vi "Process.vi"(8 "error in":errorcluster, 11 "SynchIO.USB4431":refnum<class "SynchIO.PXI-4461.lvclass">) -> (0 "error out":errorcluster, 3 "SynchIO.USB4431 out":refnum<class "SynchIO.PXI-4461.lvclass">)   [LabVIEW 2016, in "SynchIO.PXI-4461.lvclass"]
doc: "---------------------------------------------------------------\nJKI State Machine Objects™\nhttp://jki.net/state-machine-objects/\nCopyright (C) 2005-2015, JKI <info@jki.net>\nALL RIGHTS RESERVEDJKI State Machine Objects (SMO) 1.0.0.5\nJKI - JKI\nCopyright (c) 2016, JKI"
uses:
  SynchIO.PXI-4461.lvclass
  C:/Program Files/National Instruments/LabVIEW 2016/vi.lib/JKI/JKI SMO/SMO/SMO.lvclass
  <vilib>/JKI/JKI SMO/SMO/Typedefs/Parent Call--Enum.ctl
  SynchIO/SynchIO.lvclass
  <vilib>/JKI/JKI SMO/SMO/SMO.lvclass
  <resource>/objmgr/ni.dex.rc
panel:
  in  "Start":bool
  in  "stop":bool
  in  "Tab Control":T1(tab)
  in  "AI Configuration":T2(array[cluster])=[{"AI.Coupling"=enum."DC", "AI.Max"=1.0, "AI.Min"=-1.0, "Input physical channels"="PXI1Slot2/ai0:1"}, {"AI.Coupling"=enum."DC", "AI.Max"=1.0, "AI.Min"=-1.0, "Input physical channels"="PXI1Slot5/ai0:1"}, {"AI.Coupling"=enum."DC", "AI.Max"=1.0, "AI.Min"=-1.0, "Input physical channels"="PXI1Slot6/ai0:1"}]
  in  "AO Configuration":T3(array[cluster])=[{"Output physical channels"="PXI1Slot2/ao0:1", "AO. Max"=1.0, "AO.Min"=-1.0}, {"Output physical channels"="PXI1Slot5/ao0:1", "AO. Max"=1.0, "AO.Min"=-1.0}, {"Output physical channels"="PXI1Slot6/ao0:1", "AO. Max"=1.0, "AO.Min"=-1.0}]
  in  "sampling info":cluster{"Fs":dbl, "#s":dbl}={"Fs"=102388.0, "#s"=7876.0}
  in  "AI Buffer Size (S)":i32=100
  in  "AO":T4={"AO amp (V)"=[1.0, 0.0, 0.0, 0.0, 0.0, 0.0, 0.0, 0.0], "AO DC (V)"=[0.0, 0.0, 0.0, 0.0, 0.0, 0.0, 0.0, 0.0], "AO f (Hz)"=[13.0, 13.0, 13.0, 13.0, 13.0, 13.0, 13.0, 13.0], "AO phi (deg)"=[0.0, 0.0, 0.0, 0.0, 0.0, 0.0, 0.0, 0.0], "function"=[enum."Sine Wave", enum."Sine Wave", enum."Sine Wave", enum."Sine Wave", enum."Sine Wave", enum."Sine Wave", enum."Sine Wave", enum."Sine Wave"]} {"AO DC (V)" format="%#_6p"; "AO amp (V)" format="%#_6p"}
  out "Signals Graph":waveform(dbl)[](graph)=[{"t0"=timestamp(3565974471.4961195 s since 1904-01-01), "dt"=1.0, "Y"=array[6023 elements], "attributes"=variant("NI_ChannelName"=variant(string "Dev2/ai0"), "NI_UnitDescription"=variant(string "Volts"))}, {"t0"=timestamp(3565974471.4961195 s since 1904-01-01), "dt"=1.0, "Y"=array[6023 elements], "attributes"=variant("NI_ChannelName"=variant(string "Dev2/ai1"), "NI_UnitDescription"=variant(string "Volts"))}, {"t0"=timestamp(3565974471.4961195 s since 1904-01-01), "dt"=1.0, "Y"=array[6023 elements], "attributes"=variant("NI_ChannelName"=variant(string "Dev2/ai2"), "NI_UnitDescription"=variant(string "Volts"))}, {"t0"=timestamp(3565974471.4961195 s since 1904-01-01), "dt"=1.0, "Y"=array[6023 elements], "attributes"=variant("NI_ChannelName"=variant(string "Dev2/ai3"), "NI_UnitDescription"=variant(string "Volts"))}, {"t0"=timestamp(3565974471.554943 s since 1904-01-01), "dt"=1.0, "Y"=array[6023 elements], "attributes"=variant("NI_ChannelName"=variant(string "Dev2/ai0"), "NI_UnitDescription"=variant(string "Volts"))}, {"t0"=timestamp(3565974471.554943 s since 1904-01-01), "dt"=1.0, "Y"=array[6023 elements], "attributes"=variant("NI_ChannelName"=variant(string "Dev2/ai1"), "NI_UnitDescription"=variant(string "Volts"))}]
  out "Signals Graph 2":waveform(dbl)[](graph)=[{"t0"=timestamp(3565974471.4961195 s since 1904-01-01), "dt"=1.0, "Y"=array[6023 elements], "attributes"=variant("NI_ChannelName"=variant(string "Dev2/ai0"), "NI_UnitDescription"=variant(string "Volts"))}, {"t0"=timestamp(3565974471.4961195 s since 1904-01-01), "dt"=1.0, "Y"=array[6023 elements], "attributes"=variant("NI_ChannelName"=variant(string "Dev2/ai1"), "NI_UnitDescription"=variant(string "Volts"))}, {"t0"=timestamp(3565974471.4961195 s since 1904-01-01), "dt"=1.0, "Y"=array[6023 elements], "attributes"=variant("NI_ChannelName"=variant(string "Dev2/ai2"), "NI_UnitDescription"=variant(string "Volts"))}, {"t0"=timestamp(3565974471.4961195 s since 1904-01-01), "dt"=1.0, "Y"=array[6023 elements], "attributes"=variant("NI_ChannelName"=variant(string "Dev2/ai3"), "NI_UnitDescription"=variant(string "Volts"))}, {"t0"=timestamp(3565974471.554943 s since 1904-01-01), "dt"=1.0, "Y"=array[6023 elements], "attributes"=variant("NI_ChannelName"=variant(string "Dev2/ai0"), "NI_UnitDescription"=variant(string "Volts"))}, {"t0"=timestamp(3565974471.554943 s since 1904-01-01), "dt"=1.0, "Y"=array[6023 elements], "attributes"=variant("NI_ChannelName"=variant(string "Dev2/ai1"), "NI_UnitDescription"=variant(string "Volts"))}]
  out "Current State":string="Exit"
  out "State History":string
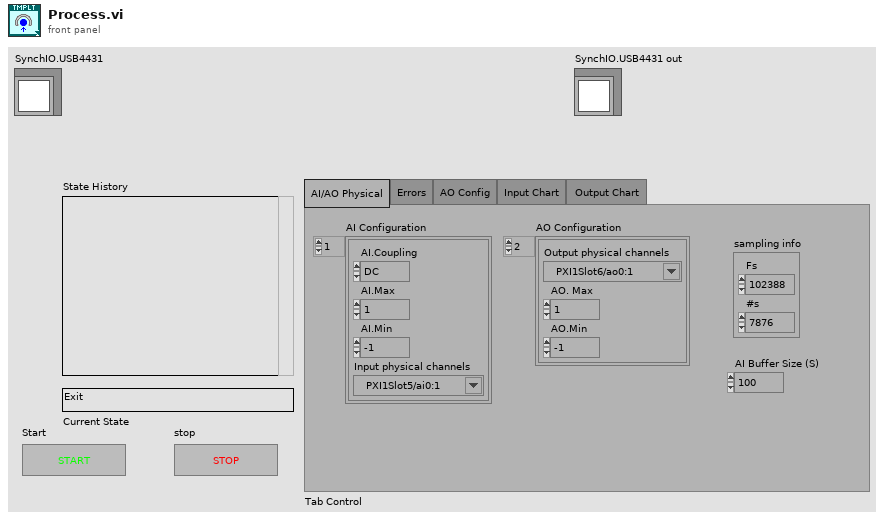
[diagram p1: front panel]
types:
  T1 = enum32{"AI/AO Physical", "Errors", "AO Config", "Input Chart", "Output Chart "}
  T2 = cluster{"AI.Coupling":enum16{"AC", "DC", "GND"}, "AI.Max":dbl, "AI.Min":dbl, "Input physical channels":tag}[]
  T3 = cluster{"Output physical channels":tag, "AO. Max":dbl, "AO.Min":dbl}[]
  T4 = cluster{"AO amp (V)":dbl[], "AO DC (V)":dbl[], "AO f (Hz)":dbl[], "AO phi (deg)":dbl[], "function":enum16{"Sine Wave", "Triangle Wave", "Square Wave", "Sawtooth Wave"}[]}
  T5 = typedef "SMO.lvclass/Parent Call--Enum.ctl" = enum16{"Allows parent to run", "Does not request parent to run"}
  T6 = enum32{"invalid app kind", "Development System", "Run Time System", "Student Edition", "Embedded LabVIEW", "Evaluation", "Custom"}
  T7 = enum32{"Invalid", "Standard", "Closed", "Hidden", "Minimized", "Maximized"}
  T8 = cluster{"Core":cluster{"Current VI Reference":refnum<vi>, "Close Panel on Exit?":bool, "error":errorcluster}, "Self Reference":refnum<class "SynchIO.PXI-4461.lvclass">, "Your string data":string, "AI Buffer Size (S)":i32, "AI Configuration":cluster{"AI.Coupling":enum16{"AC", "DC", "GND"}, "AI.Max":dbl, "AI.Min":dbl, "Input physical channels":tag}[], "AO Configuration":cluster{"Output physical channels":tag, "AO. Max":dbl, "AO.Min":dbl}[], "sampling info":cluster{"Fs":dbl, "#s":dbl}, "AI task":refnum<k21>[], "AO Task":refnum<k21>[], "AI Data":waveform(dbl)[], "AO Data":waveform(dbl)[], "AO":cluster{"AO amp (V)":dbl[], "AO DC (V)":dbl[], "AO f (Hz)":dbl[], "AO phi (deg)":dbl[], "function":enum16{"Sine Wave", "Triangle Wave", "Square Wave", "Sawtooth Wave"}[]}, "Iteration":i32, "writer endpoint":refnum<k21>, "reader endpoint":refnum<k21>, "url":string}
  T9 = cluster{"Current VI Reference":refnum<vi>, "Close Panel on Exit?":bool, "error":errorcluster}
  T10 = typedef "SMO.lvclass/Protected Events.ctl" = cluster{"StopProcesses":refnum<user-event>, "AbortProcesses":refnum<user-event>, "Config Changed":refnum<user-event>, "Dependency":refnum<user-event>}
  T11 = typedef "SynchIO.PXI-4461.lvclass/ProtectedEvents--Cluster.ctl" = cluster{"API_Template":refnum<user-event>}
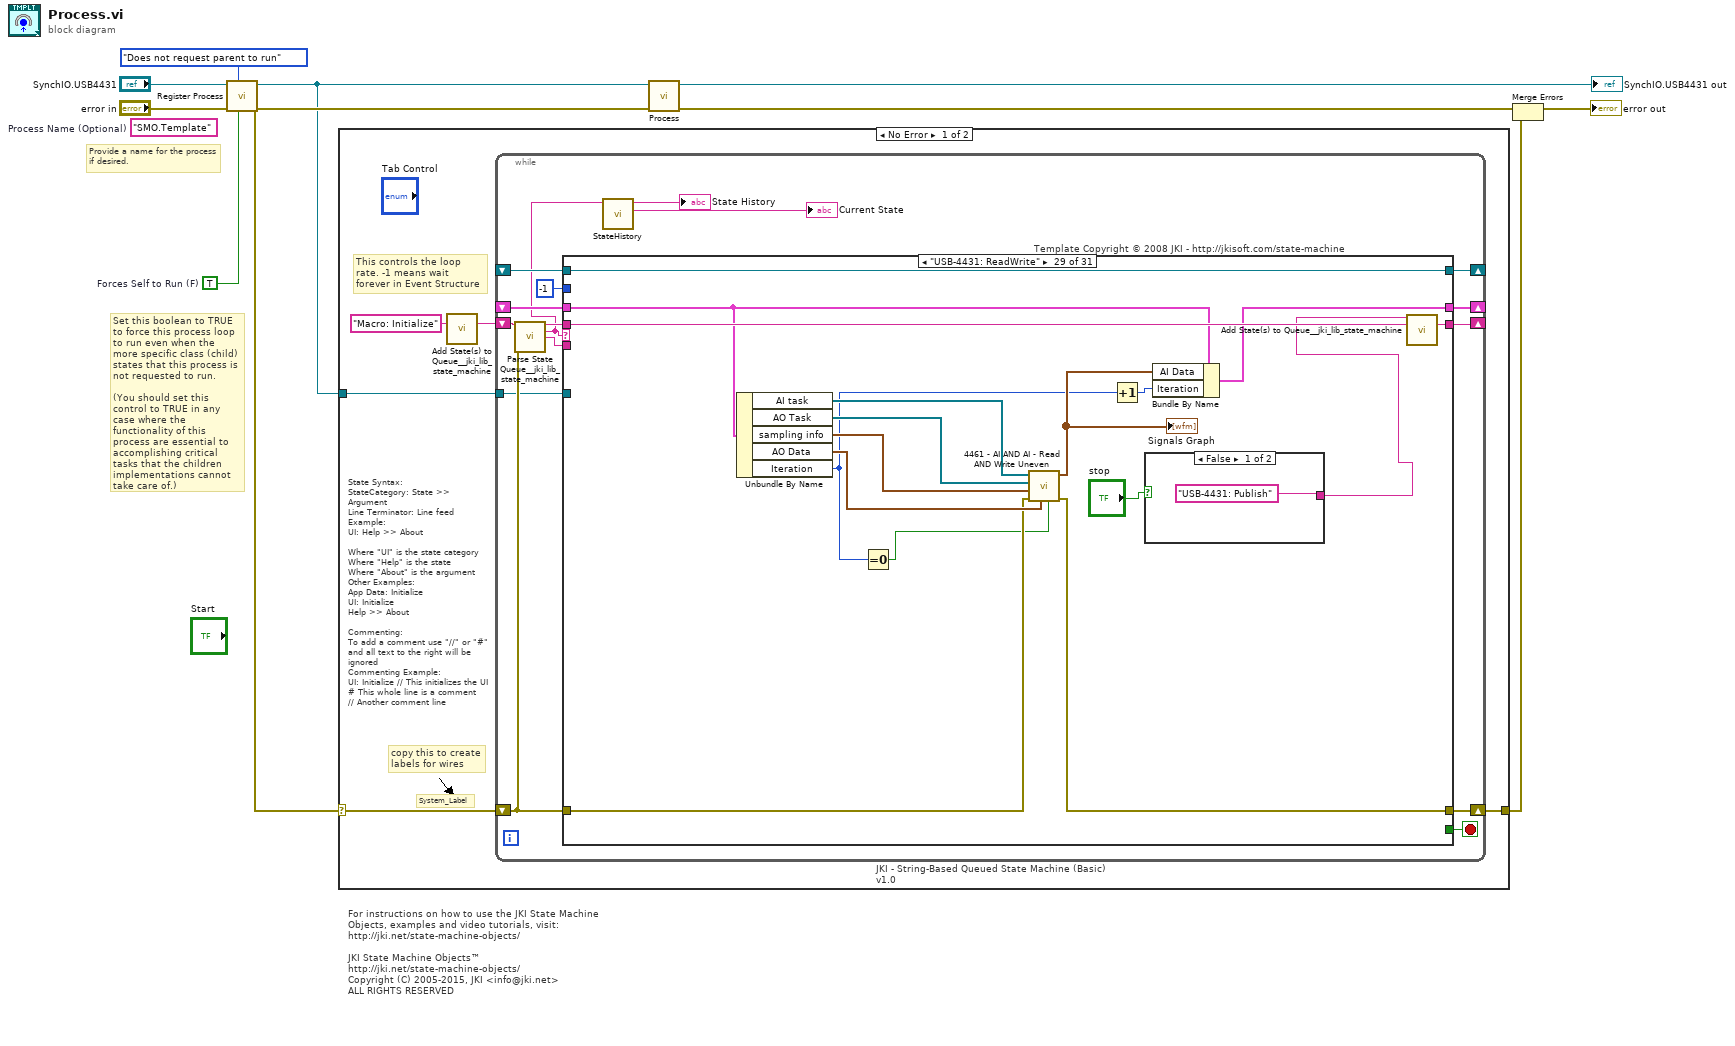
[diagram p0: block diagram]
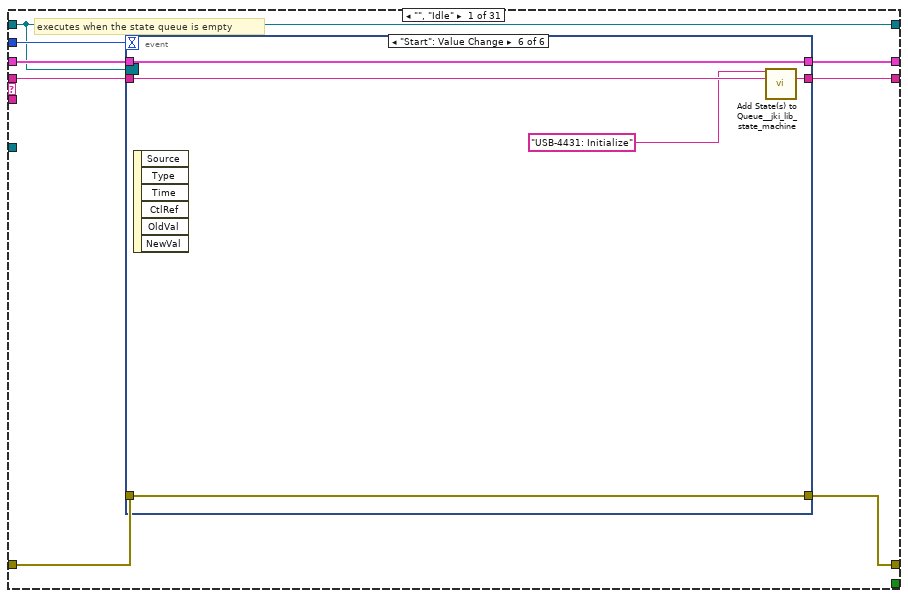
[diagram p2: hidden frame]
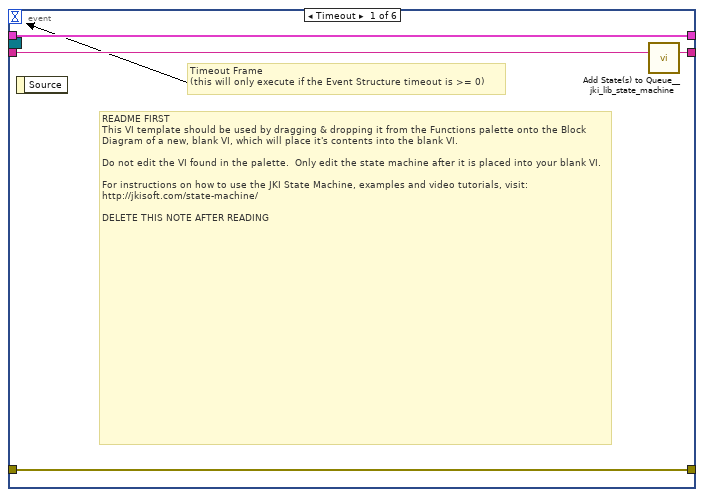
[diagram p3: hidden frame]
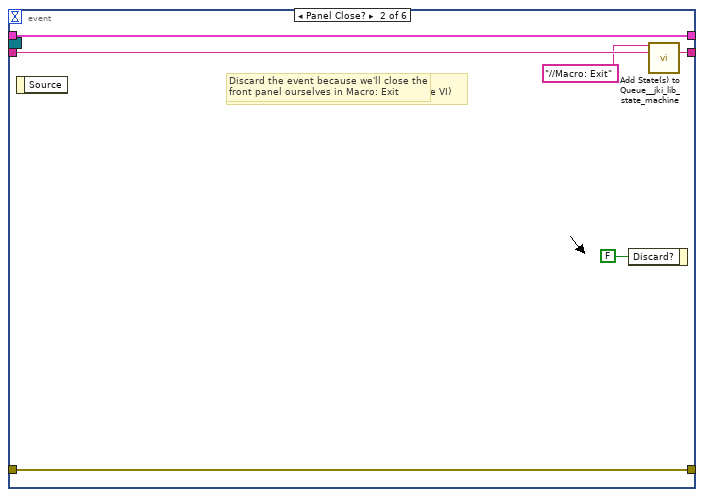
[diagram p4: hidden frame]
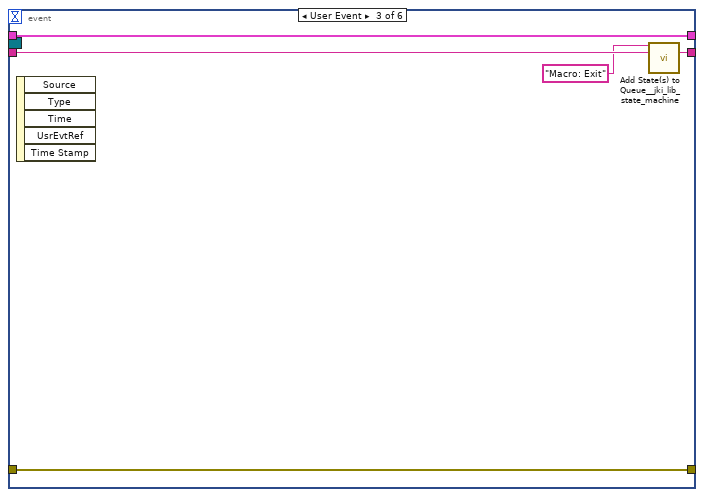
[diagram p5: hidden frame]
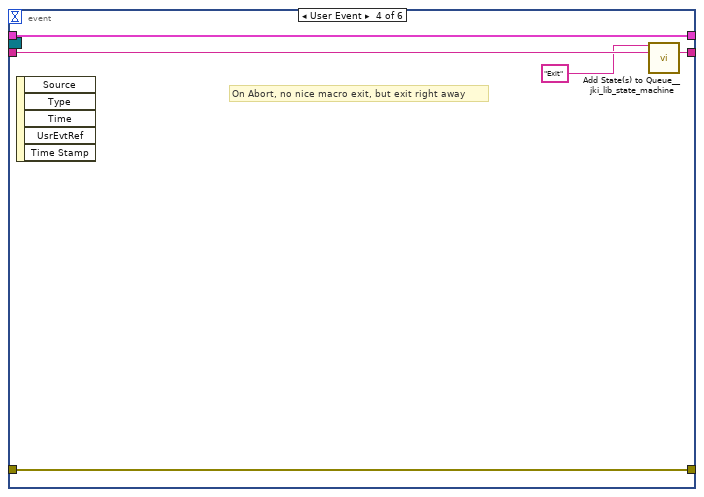
[diagram p6: hidden frame]
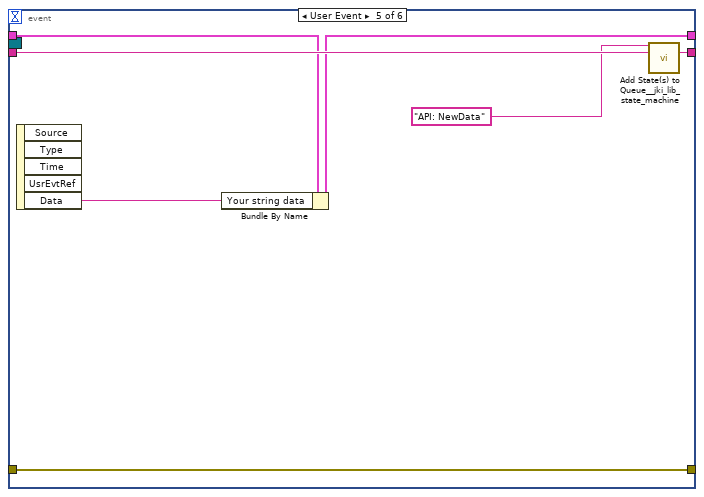
[diagram p7: hidden frame]
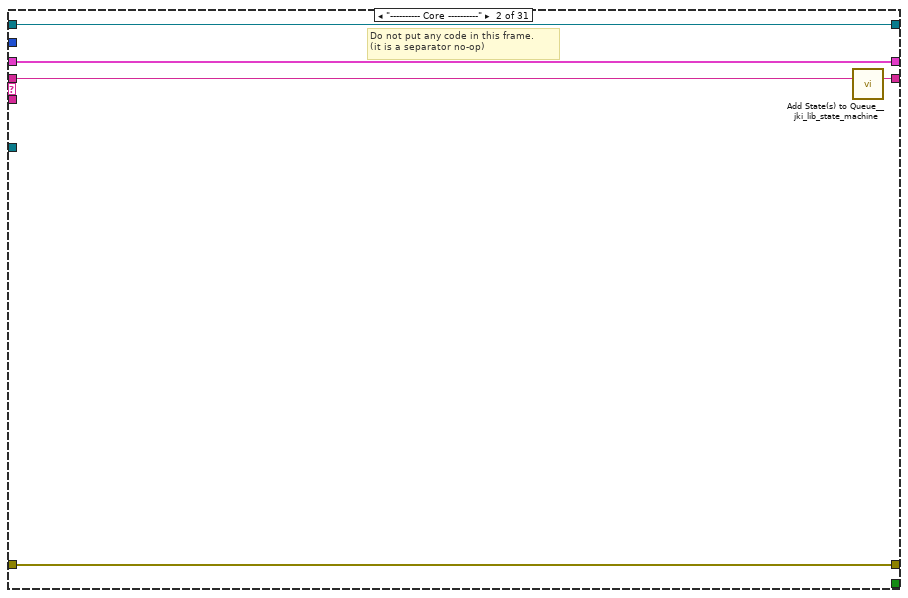
[diagram p8: hidden frame]
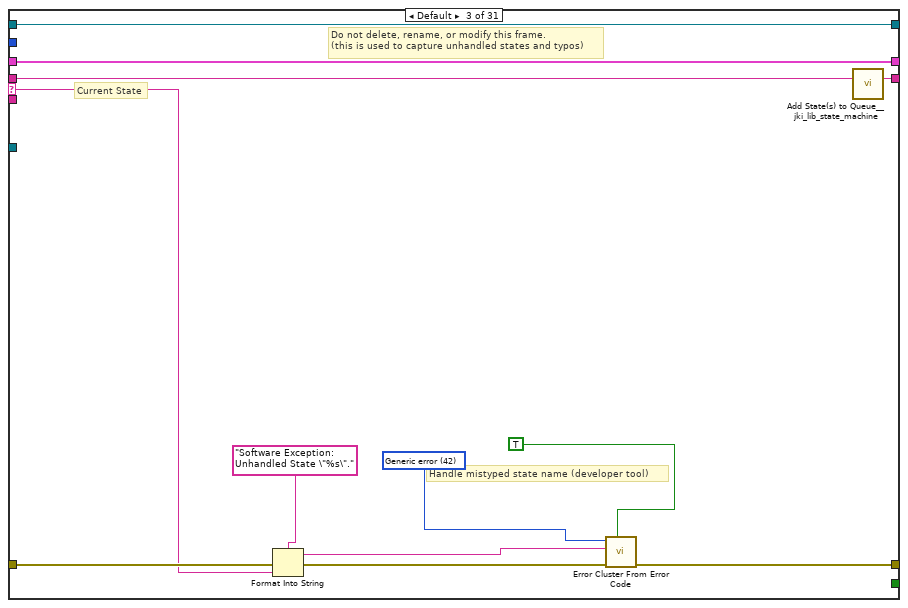
[diagram p9: hidden frame]
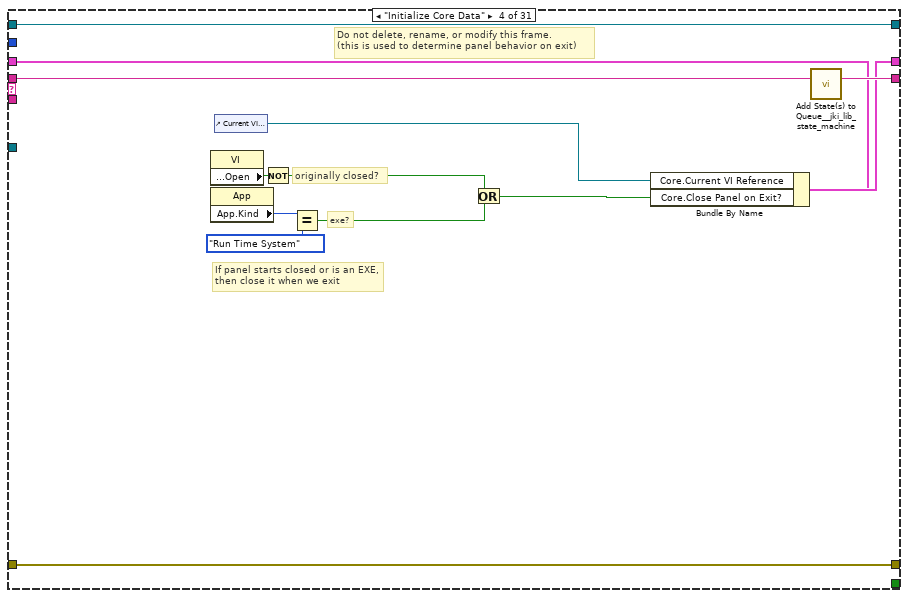
[diagram p10: hidden frame]
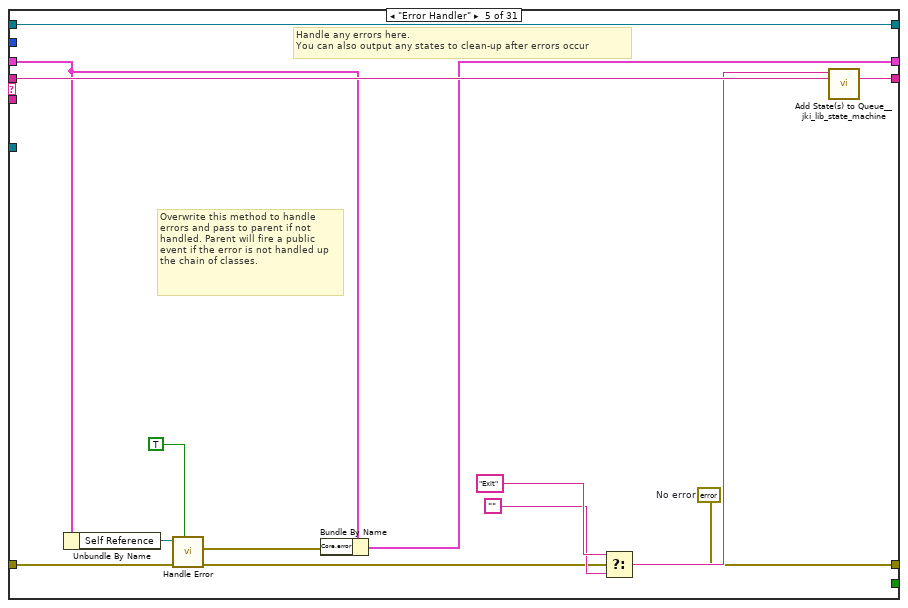
[diagram p11: hidden frame]
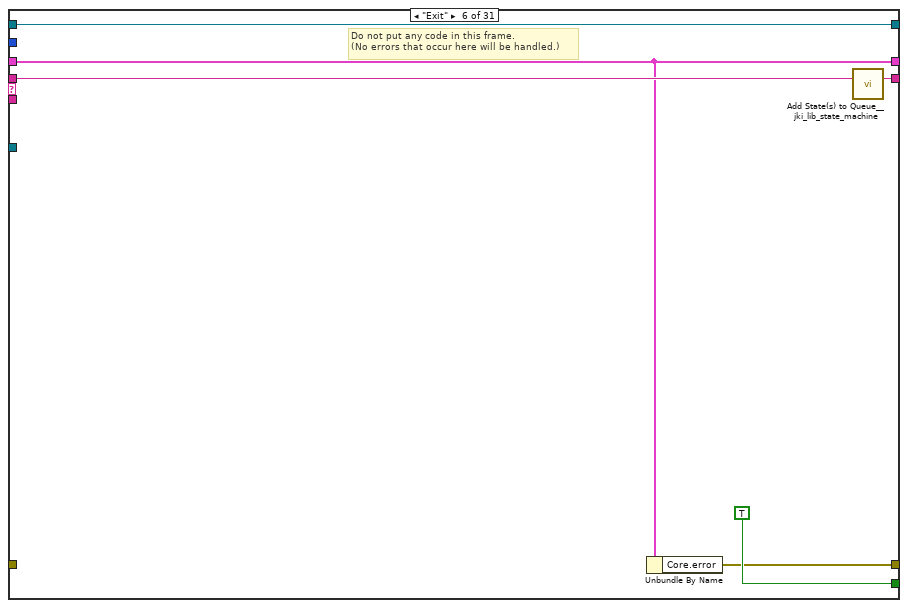
[diagram p12: hidden frame]
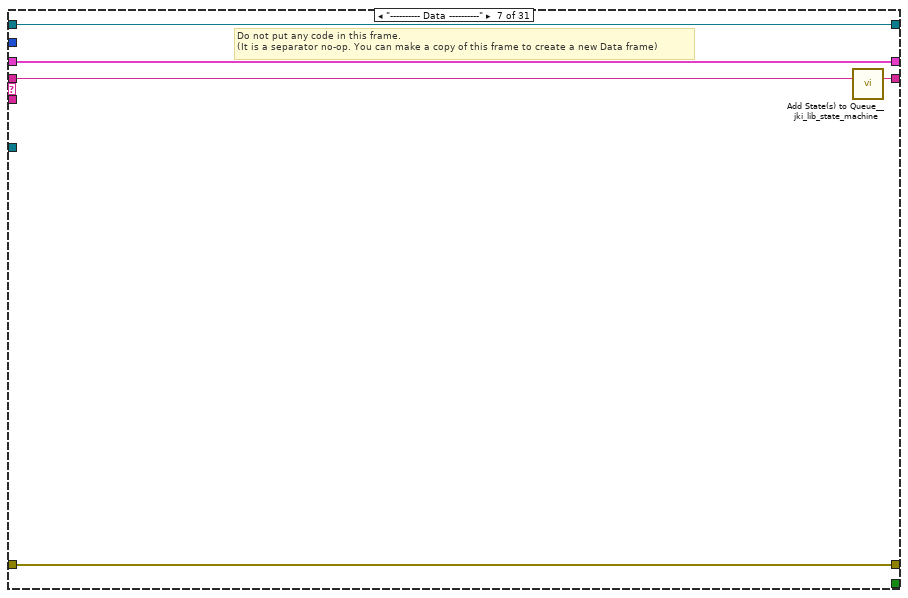
[diagram p13: hidden frame]
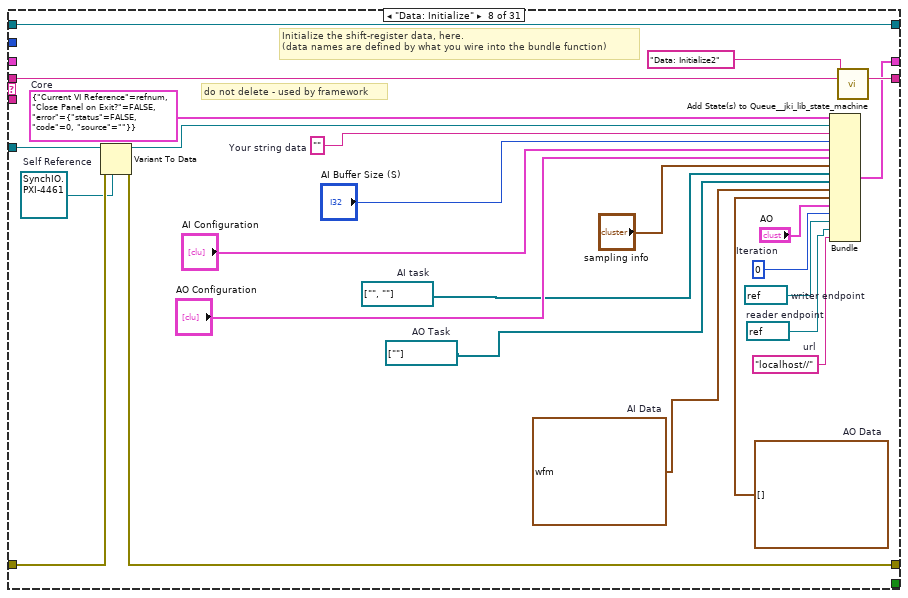
[diagram p14: hidden frame]
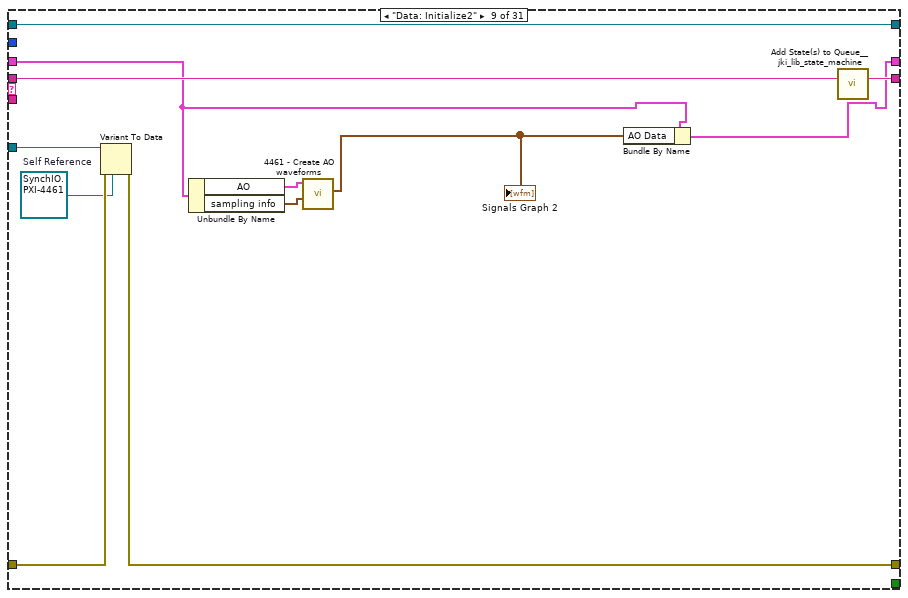
[diagram p15: hidden frame]
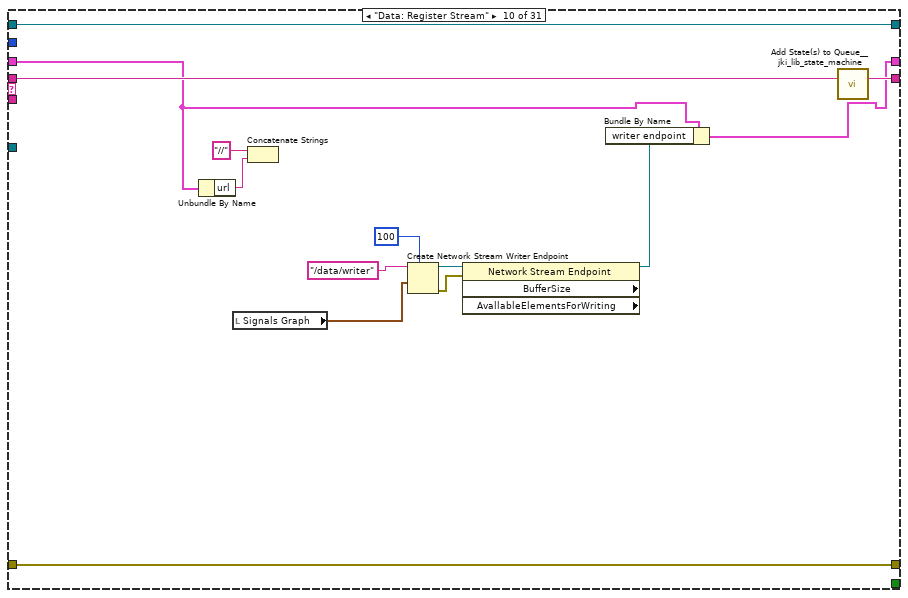
[diagram p16: hidden frame]
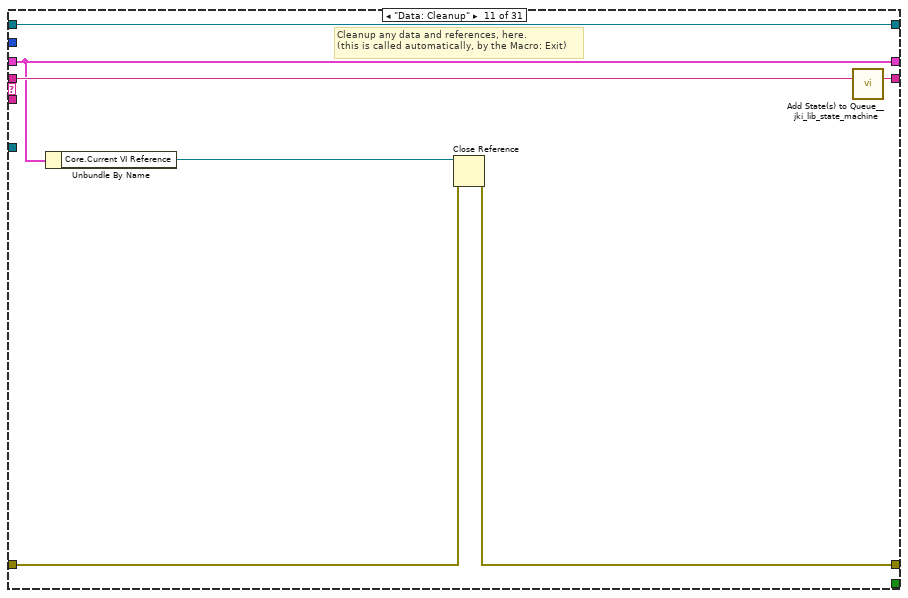
[diagram p17: hidden frame]
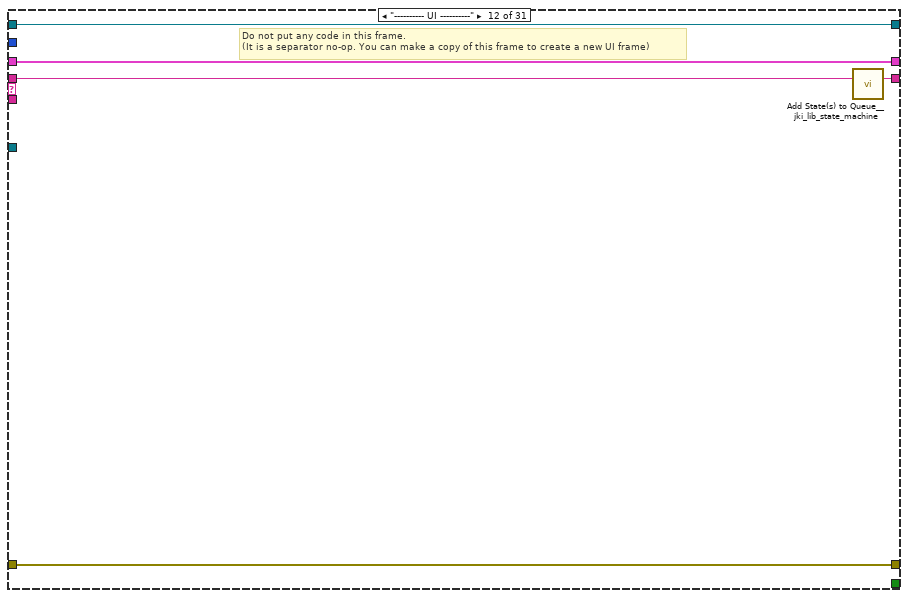
[diagram p18: hidden frame]
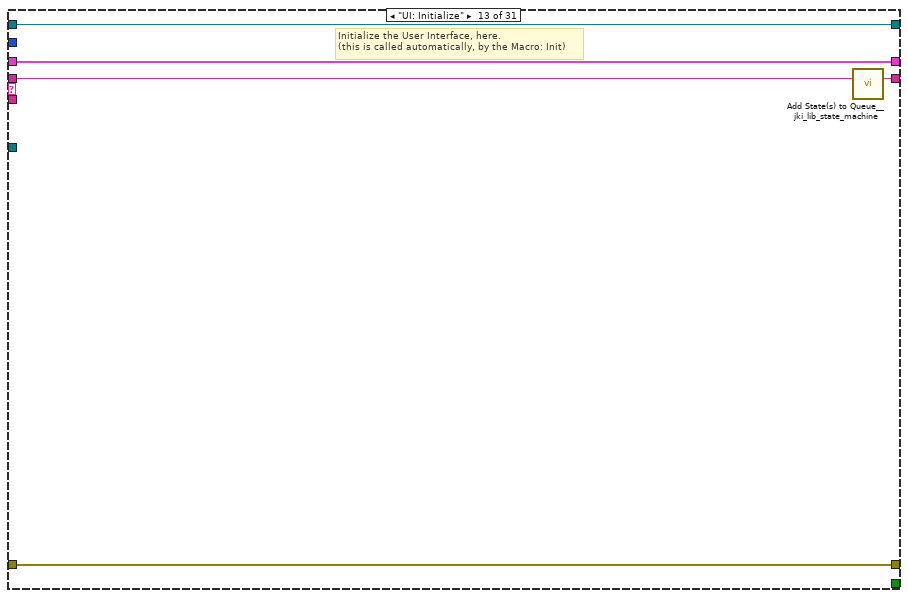
[diagram p19: hidden frame]
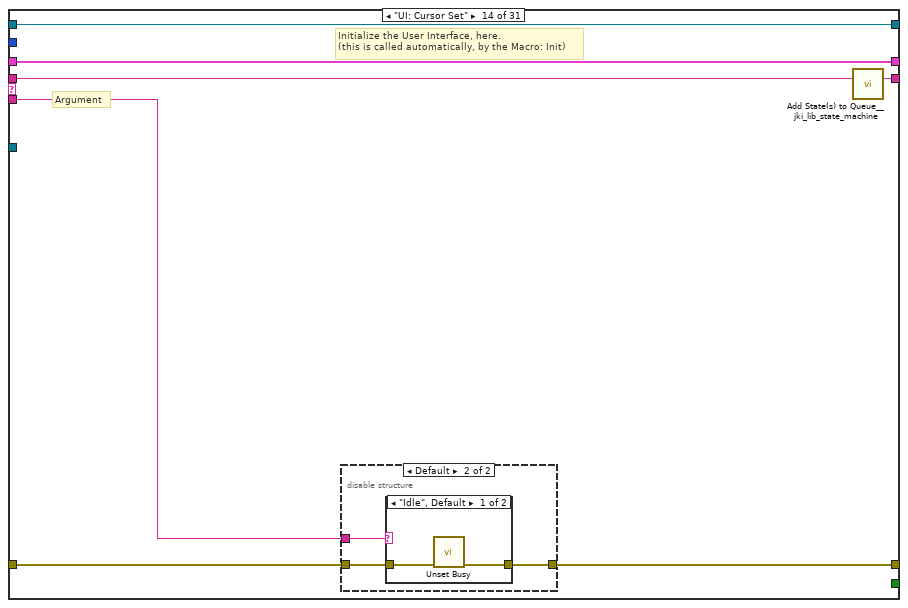
[diagram p20: hidden frame]
diagram:
  w1 = TRUE  # Forces Self to Run (F)
  (unwired) "SMO.Template"  # Process Name (Optional)
  # "Provide a name for the process\nif desired."
  # "Set this boolean to TRUE to force this process loop to run even when the more specific class (child) states that this process is not requested to run.\n\n(You should set this control to TRUE in any case where the functionality of this process are essential to accomplishing critical tasks that the children implementations cannot take care of.)"
  # "For instructions on how to use the JKI State Machine Objects, examples and video tutorials, visit:\nhttp://jki.net/state-machine-objects/\n\nJKI State Machine Objects™\nhttp://jki.net/state-machine-objects/\nCopyright (C) 2005-2015, JKI <info@jki.net>\nALL RIGHTS RESERVED"
  n1 = call <vilib>:"Register Process.vi"("Forces Self to Run (F)"=w1, "Parent Call"=Parent_Call--Enum."Does not request parent to run", "error in (no error)"="error in", "SMO"="SynchIO.USB4431") -> ("error out"=w7:errorcluster, "SMO out"=w6:refnum<class "SynchIO.PXI-4461.lvclass">)  [unwired: 6 in]
  n2 = case shown="No Error" w7 {
    selector: w7 -> [w12 w411]
    tunnel: w6 -> [w13 _]
    tunnel: [w11 w411] -> w3
    frame No Error {
      # "State Syntax:\nStateCategory: State >> Argument\nLine Terminator: Line feed\nExample:\nUI: Help >> About\n\nWhere \"UI\" is the state category\nWhere \"Help\" is the state\nWhere \"About\" is the argument\nOther Examples:\nApp Data: Initialize\nUI: Initialize\nHelp >> About\n\nCommenting:\nTo add a comment use \"//\" or \"#\" and all text to the right will be ignored\nCommenting Example:\nUI: Initialize // This initializes the UI\n# This whole line is a comment\n// Another comment line"
      # "copy this to create labels for wires"
      # "This controls the loop rate. -1 means wait forever in Event Structure"
      # "System_Label"
      n3 = call <vilib>:"Add State(s) to Queue__jki_lib_state_machine.vi"("State(s) in (\"\")"="Macro: Initialize") -> ("States Out"=w15:string)  [unwired: 14 in]
      n4 = while "JKI - String-Based Queued State Machine (Basic) v1.0" {
        shift-right: [w26] -> _
        shift-left: _ -> [w25]
        shift-right: [w29] -> w11
        shift-left: w12 -> [w23]
        shift-right: [w28] -> _
        shift-left: w15 -> [w30]
        tunnel: w13 -> [w22]
        shift-right: [w21] -> _
        shift-left: _ -> [w20]
        stop <- w27 stop-if-true
        # "Template Copyright © 2008 JKI - http://jkisoft.com/state-machine"
        n5 = call <vilib>:"Parse State Queue__jki_lib_state_machine.vi"("State Queue"=w30, "Error In (no error)"=w23) -> ("Remaining States"=w17:string, "Current State"=w16:string, "Arguments"=w31:string)  [unwired: 11 in]
        n6 = case shown="\"USB-4431: ReadWrite\"" w16 {
          selector: w16 -> [_ _ w78 _ _ _ _ _ _ _ _ _ _ _ _ _ _ _ _ _ _ _ _ _ _ _ _ _ _ _ _]
          tunnel: w17 -> [w39 w76 w82 w101 w115 w121 w126 w151 w163 w177 w184 w189 w194 w201 w217 w249 w258 w272 w277 w288 w298 w311 w317 w322 w330 w335 w340 w356 w373 w385 w397]
          tunnel: w31 -> [_ _ _ _ _ _ _ _ _ _ _ _ _ w195 w211 _ _ _ _ _ _ _ _ _ _ _ _ _ _ _ _]
          tunnel: w25 -> [w37 w73 w80 w92 w104 w117 w123 _ w154 w174 w179 w186 w192 w199 w213 w246 w254 w263 w274 w285 w295 w309 w315 w320 w327 w332 w338 w349 w370 w382 w392]
          tunnel: [w36 w74 w84 w98 w106 w116 w124 w146 w160 w167 w180 w187 w191 w196 w214 w247 w256 w270 w275 w279 w296 w299 w313 w318 w324 w331 w336 w345 w365 w379 w394] -> w29
          tunnel: w23 -> [w35 w74 w83 w98 w111 _ w124 w147 w161 w167 w181 w187 w191 w197 w215 w247 w256 w270 w275 w280 w296 w303 w313 w318 w325 w331 w336 w346 w360 w379 w393]
          tunnel: [w38 w75 w81 w100 w114 w120 w125 w150 w162 w176 w183 w188 w193 w200 w216 w248 w257 w271 w276 w287 w297 w310 w316 w321 w329 w334 w339 w355 w372 w384 w396] -> w28
          tunnel: [_ _ _ _ _ TRUE _ _ _ _ _ _ _ _ _ _ _ _ _ _ _ _ _ _ _ _ _ _ _ _ _] -> w27
          tunnel: [w34 w73 w80 w99 w103 w117 w123 w149 w153 w173 w179 w186 w192 w199 w213 w246 w254 w263 w274 w285 w295 w309 w315 w320 w327 w332 w338 w348 w369 w381 w392] -> w26
          tunnel: -1 ("Timeout") -> [w33 _ _ _ _ _ _ _ _ _ _ _ _ _ _ _ _ _ _ _ _ _ _ _ _ _ _ _ _ _ _]
          tunnel: w22 -> [_ _ _ _ _ _ _ w144 w158 _ _ _ _ _ _ _ _ _ _ _ _ _ _ _ _ _ _ _ _ _ _]
          tunnel: [w32 w72 w77 w89 w113 w118 w122 w142 w157 w175 w178 w185 w190 w198 w210 w245 w255 w264 w273 w286 w294 w308 w314 w319 w328 w333 w337 w354 w371 w383 w395] -> w21
          tunnel: w20 -> [w32 w72 w77 w89 w113 w118 w122 w142 w157 w175 w178 w185 w190 w198 w210 w245 w255 w264 w273 w286 w294 _ w314 w319 w328 w333 w337 w354 w371 w383 w395]
          frame "", "Idle" {
            # "executes when the state queue is empty"
            n7 = event shown="[5] \"Start\": Value Change" {
              selector: w32 -> [_ _ _ _ _ _]
              dyn-events: _ -> [_ _ _ _ _ _]
              timeout: w33 -> [_ _ _ _ _ _]
              tunnel: w39 -> [w43 w49 w54 w59 w66 w71]
              tunnel: [w42 w48 w53 w58 w65 w70] -> w38
              tunnel: w37 -> [w40 w46 w51 w56 w63 w67]
              tunnel: [w41 w47 w52 w57 w64 w69] -> w36
              tunnel: w35 -> [w41 w47 w52 w57 w64 w69]
              tunnel: [w40 w46 w51 w56 w62 w67] -> w34
              event Timeout {
                # "README FIRST\nThis VI template should be used by dragging & dropping it from the Functions palette onto the Block Diagram of a new, blank VI, which will place it's contents into the blank VI.\n\nDo not edit the VI found in the palette.  Only edit the state machine after it is placed into your blank VI.\n\nFor instructions on how to use the JKI State Machine, examples and video tutorials, visit:\nhttp://jkisoft.com/state-machine/\n\nDELETE THIS NOTE AFTER READING"
                # "Timeout Frame\n(this will only execute if the Event Structure timeout is >= 0)"
                n8 = event-data() -> ()  [unwired: 1 in, 1 out]
                n9 = call <vilib>:"Add State(s) to Queue__jki_lib_state_machine.vi"("State(s) in (\"\")"=w43) -> ("States Out"=w42:string)  [unwired: 14 in]
              }
              event Panel Close? {
                # "Discard the event because we'll close the front panel ourselves in Macro: Exit"
                # "Close Panel button (pressed) Event\n(this executes Macro: Exit to terminate the VI)"
                n10 = event-data() -> ()  [unwired: 1 in, 1 out]
                n11 = event-data("Discard?"=FALSE) -> ()  [unwired: 1 in, 1 out]
                n12 = call <vilib>:"Add State(s) to Queue__jki_lib_state_machine.vi"("State(s) in Front (\"\")"="//Macro: Exit", "State(s) in (\"\")"=w49) -> ("States Out"=w48:string)  [unwired: 13 in]
              }
              event User Event {
                n13 = event-data() -> ()  [unwired: 1 in, 5 out]
                n14 = call <vilib>:"Add State(s) to Queue__jki_lib_state_machine.vi"("State(s) in Front (\"\")"="Macro: Exit", "State(s) in (\"\")"=w54) -> ("States Out"=w53:string)  [unwired: 13 in]
              }
              event User Event {
                # "On Abort, no nice macro exit, but exit right away"
                n15 = event-data() -> ()  [unwired: 1 in, 5 out]
                n16 = call <vilib>:"Add State(s) to Queue__jki_lib_state_machine.vi"("State(s) in Front (\"\")"="Exit", "State(s) in (\"\")"=w59) -> ("States Out"=w58:string)  [unwired: 13 in]
              }
              event User Event {
                n17 = event-data() -> ("Data"=w60:string)  [unwired: 1 in, 4 out]
                n18 = Bundle By Name(cluster=w63, "Your string data"=w60) -> (w62:T8)
                n19 = call <vilib>:"Add State(s) to Queue__jki_lib_state_machine.vi"("State(s) in Front (\"\")"="API: NewData", "State(s) in (\"\")"=w66) -> ("States Out"=w65:string)  [unwired: 13 in]
              }
              event "Start": Value Change {
                n20 = event-data() -> ()  [unwired: 1 in, 6 out]
                n21 = call <vilib>:"Add State(s) to Queue__jki_lib_state_machine.vi"("State(s) in Front (\"\")"="USB-4431: Initialize", "State(s) in (\"\")"=w71) -> ("States Out"=w70:string)  [unwired: 13 in]
              }
            }
          }
          frame "---------- Core ----------" {
            # "Do not put any code in this frame.\n(it is a separator no-op)"
            n22 = call <vilib>:"Add State(s) to Queue__jki_lib_state_machine.vi"("State(s) in (\"\")"=w76) -> ("States Out"=w75:string)  [unwired: 14 in]
          }
          frame Default {
            w87 = 42 items=["No error", "Argument error", "Memory is full", "Out of zone", "End of file", "File already open", "Generic file I/O error", "File not found", "File permission error", "Disk is full", "Duplicate path", "Too many files open", "System feature not enabled", "Resource file not found", "Cannot add resource", "Resource not found", "Image not found", "Image memory error", "Pen does not exist", "Config type invalid", "Config token not found", "Config parse error", "Config memory error", "Bad external code format", "Bad external code offset", "External code not present", "Null window", "Destroy window error", "Null menu", "Print aborted", "Bad print record", "Print driver error", "Windows error during printing", "Memory error during printing", "Print dialog error", "Generic print error", "Invalid device refnum", "Device not found", "Device parameter error", "Device unit error", "Cannot open device", "Device call aborted", "Generic error", "Cancelled by user", "Object ID too low", "Object ID too high", "Object not in heap", "Unknown heap", "Unknown object (invalid DefProc)", "Unknown object (DefProc not in table)", "Message out of range", "Invalid (null) method", "Unknown message", "Manager call not supported", "Bad address", "Network operation in progress", "Network operation timed out", "Connection is busy", "Network attribute not supported", "Network error", "Address in use", "System out of memory", "Connection aborted", "Connection refused", "Not connected", "Already connected", "Connection closed", "Initialization error (interapplication manager)", "Bad occurrence", "Wait on unbound occurrence handler", "Occurrence queue overflow", "Datalog type conflict", "Unused", "Unrecognized type (interapplication manager)", "Memory corrupt", "Failed to make temporary DLL", "Old CIN version", "Drag socket not found", "Failed to load drop-object", "Failed to register OLE object", "Failed to release OLE object", "Format specifier type mismatch", "Unknown format specifier", "Too few format specifiers", "Too many format specifiers", "Scan failed", "Newer CIN version", "Error converting to variant", "Runtime menu error", "Password tampered", "Variant attribute not found", "Incompatible variant data type", "Event data is not available", "Event Store is not present", "Occurrence is not found", "Event Queue is not created", "Event info is not available", "Refnum passed is NULL", "Error retrieving Class GUID", "Error retrieving CoClass GUID", "Error retrieving TypeLib GUID.", "Bad built application magic bytes.", "Specific driver is different from the specific driver associated with the Logical Name.", "There is no session opened to the class driver.", "Max Error", "MAX - Error with config objects", "MAX - Error loading configuration", "MAX - Group not supported"]
            # "Current State"
            # "Do not delete, rename, or modify this frame.\n(this is used to capture unhandled states and typos)"
            # "Handle mistyped state name (developer tool)"
            n23 = Format Into String(format string="Software Exception: Unhandled State \"%s\"." ("message"), error in=w83, w78) -> (resulting string=w86:string, error out=w85:errorcluster)  [unwired: 1 in]
            n24 = call <vilib>:"Error Cluster From Error Code.vi"("show call chain? (False)"=TRUE, "error in (no error)"=w85, "error message (\"\")"=w86, "error code (0)"=w87) -> ("error out"=w84:errorcluster)  [unwired: 5 in]
            n25 = call <vilib>:"Add State(s) to Queue__jki_lib_state_machine.vi"("State(s) in (\"\")"=w82) -> ("States Out"=w81:string)  [unwired: 14 in]
          }
          frame "Initialize Core Data" {
            # "Do not delete, rename, or modify this frame.\n(this is used to determine panel behavior on exit)"
            # "originally closed?"
            # "exe?"
            # "If panel starts closed or is an EXE, then close it when we exit"
            n26 = property class="VI"() -> ("Front Panel.Open"=w97:bool)  [unwired: 2 in, 2 out]
            n27 = property class="App"() -> ("App.Kind"=w96:T6)  [unwired: 2 in, 2 out]
            n28 = control-ref of="Current VI Reference"() -> (w90:refnum<vi>)
            n29 = Not(x=w97) -> (.not. x?=w94:bool)
            n30 = Equal?(x=w96, y=T6."Run Time System" ("Application:Kind")) -> (x = y?=w93:bool)
            n31 = Or(x=w94, y=w93) -> (x .or. y?=w91:bool)
            n32 = Bundle By Name(cluster=w92, "Core.Current VI Reference"=w90, "Core.Close Panel on Exit?"=w91) -> (w99:T8)
            n33 = call <vilib>:"Add State(s) to Queue__jki_lib_state_machine.vi"("State(s) in (\"\")"=w101) -> ("States Out"=w100:string)  [unwired: 14 in]
          }
          frame "Error Handler" {
            w106 = errorcluster {"status"=FALSE, "code"=0, "source"=""}  # No error
            # "Overwrite this method to handle errors and pass to parent if not handled. Parent will fire a public event if the error is not handled up the chain of classes."
            # "Handle any errors here.\nYou can also output any states to clean-up after errors occur"
            n34 = Unbundle By Name(w104) -> ("Self Reference"=w112:refnum<class "SynchIO.PXI-4461.lvclass">)
            n35 = call-dynamic "Handle Error.vi"("Stop on Unhandled Error (T)"=TRUE, "error in"=w111, "SMO"=w112) -> ("handling error"=w107:errorcluster, "Unhandled error"=w105:errorcluster)  [unwired: 6 in, 1 out]
            n36 = Bundle By Name(cluster=w104, "Core.error"=w105) -> (w103:T8)
            n37 = Select(t="Exit", s=w107, f="") -> (s? t:f=w108:string)
            n38 = call <vilib>:"Add State(s) to Queue__jki_lib_state_machine.vi"("State(s) in Front (\"\")"=w108, "State(s) in (\"\")"=w115) -> ("States Out"=w114:string)  [unwired: 13 in]
          }
          frame "Exit" {
            # "Do not put any code in this frame.\n(No errors that occur here will be handled.)"
            n39 = Unbundle By Name(w117) -> ("Core.error"=w116:errorcluster)
            n40 = call <vilib>:"Add State(s) to Queue__jki_lib_state_machine.vi"("State(s) in (\"\")"=w121) -> ("States Out"=w120:string)  [unwired: 14 in]
          }
          frame "---------- Data ----------" {
            # "Do not put any code in this frame.\n(It is a separator no-op. You can make a copy of this frame to create a new Data frame)"
            n41 = call <vilib>:"Add State(s) to Queue__jki_lib_state_machine.vi"("State(s) in (\"\")"=w126) -> ("States Out"=w125:string)  [unwired: 14 in]
          }
          frame "Data: Initialize" {
            w127 = "localhost//"  # url
            w128 = refnum<k21> refnum  # reader endpoint
            w129 = waveform(dbl)[] [{"t0"=timestamp(3565974471.4961195 s since 1904-01-01), "dt"=1.0, "Y"=array[6023 elements], "attributes"=variant("NI_ChannelName"=variant(string "Dev2/ai0"), "NI_UnitDescription"=variant(string "Volts"))}, {"t0"=timestamp(3565974471.4961195 s since 1904-01-01), "dt"=1.0, "Y"=array[6023 elements], "attributes"=variant("NI_ChannelName"=variant(string "Dev2/ai1"), "NI_UnitDescription"=variant(string "Volts"))}, {"t0"=timestamp(3565974471.4961195 s since 1904-01-01), "dt"=1.0, "Y"=array[6023 elements], "attributes"=variant("NI_ChannelName"=variant(string "Dev2/ai2"), "NI_UnitDescription"=variant(string "Volts"))}, {"t0"=timestamp(3565974471.4961195 s since 1904-01-01), "dt"=1.0, "Y"=array[6023 elements], "attributes"=variant("NI_ChannelName"=variant(string "Dev2/ai3"), "NI_UnitDescription"=variant(string "Volts"))}, {"t0"=timestamp(3565974471.554943 s since 1904-01-01), "dt"=1.0, "Y"=array[6023 elements], "attributes"=variant("NI_ChannelName"=variant(string "Dev2/ai0"), "NI_UnitDescription"=variant(string "Volts"))}, {"t0"=timestamp(3565974471.554943 s since 1904-01-01), "dt"=1.0, "Y"=array[6023 elements], "attributes"=variant("NI_ChannelName"=variant(string "Dev2/ai1"), "NI_UnitDescription"=variant(string "Volts"))}]  # AI Data
            w130 = refnum<k21> refnum  # writer endpoint
            w131 = 0  # Iteration
            w133 = waveform(dbl)[] []  # AO Data
            w134 = refnum<k21>[] [""]  # AO Task
            w135 = refnum<k21>[] ["", ""]  # AI task
            w141 = T9 {"Current VI Reference"=refnum, "Close Panel on Exit?"=FALSE, "error"={"status"=FALSE, "code"=0, "source"=""}}  # Core
            w145 = refnum<class "SynchIO.PXI-4461.lvclass"> refnum  # Self Reference
            w148 = ""  # Your string data
            # "do not delete - used by framework"
            # "Initialize the shift-register data, here.\n(data names are defined by what you wire into the bundle function)"
            n42 = Variant To Data(error in=w147, type=w145, Variant=w144) -> (data=w143:refnum<class "SynchIO.PXI-4461.lvclass">, error out=w146:errorcluster)
            n43 = Bundle("Core"=w141, "Self Reference"=w143, "Your string data"=w148, "AI Buffer Size (S)"="AI Buffer Size (S)", "AI Configuration"="AI Configuration", "AO Configuration"="AO Configuration", "sampling info"="sampling info", "AI task"=w135, "AO Task"=w134, "AI Data"=w129, "AO Data"=w133, "AO"="AO", "Iteration"=w131, "writer endpoint"=w130, "reader endpoint"=w128, "url"=w127) -> (w149:T8)  [unwired: 1 in]
            n44 = call <vilib>:"Add State(s) to Queue__jki_lib_state_machine.vi"("State(s) in Front (\"\")"="Data: Initialize2" ("State(s) in Front (\"\")"), "State(s) in (\"\")"=w151) -> ("States Out"=w150:string)  [unwired: 13 in]
          }
          frame "Data: Initialize2" {
            w159 = refnum<class "SynchIO.PXI-4461.lvclass"> refnum  # Self Reference
            n45 = Variant To Data(error in=w161, type=w159, Variant=w158) -> (error out=w160:errorcluster)  [unwired: 1 out]
            n46 = Unbundle By Name(w154) -> ("AO"=w155:T4, "sampling info"=w156:cluster{"Fs":dbl, "#s":dbl})
            n47 = call "4461 - Create AO waveforms.vi"("sampling info"=w156, "AO"=w155) -> ("AO Array"=w152:waveform(dbl)[])  [unwired: 6 in, 3 out]
            "Signals Graph 2" <- w152
            n48 = Bundle By Name(cluster=w154, "AO Data"=w152) -> (w153:T8)
            n49 = call <vilib>:"Add State(s) to Queue__jki_lib_state_machine.vi"("State(s) in (\"\")"=w163) -> ("States Out"=w162:string)  [unwired: 14 in]
          }
          frame "Data: Register Stream" {
            n50 = Unbundle By Name(w174) -> ("url"=w164:string)
            n51 = local read "Signals Graph"() -> (w166:waveform(dbl)[])
            n52 = Concatenate Strings("//" ("reader url"), w164) -> ()  [unwired: 1 out]
            n53 = Create Network Stream Writer Endpoint(7:100 ("writer buffer size"), 9:w166, 11:"/data/writer" ("reader url")) -> (0:w170:errorcluster, 3:w171:refnum<k21>)  [unwired: 4 in]
            n54 = property class="Network Stream Endpoint" props=["BufferSize", "AvallableElementsForWriting"](reference=w171, error in=w170) -> (reference out=w168:refnum<k21>)  [unwired: 3 out]
            n55 = Bundle By Name(cluster=w174, "writer endpoint"=w168) -> (w173:T8)
            n56 = call <vilib>:"Add State(s) to Queue__jki_lib_state_machine.vi"("State(s) in (\"\")"=w177) -> ("States Out"=w176:string)  [unwired: 14 in]
          }
          frame "Data: Cleanup" {
            # "Cleanup any data and references, here.\n(this is called automatically, by the Macro: Exit)"
            n57 = Unbundle By Name(w179) -> ("Core.Current VI Reference"=w182:refnum<vi>)
            n58 = Close Reference(reference=w182, error in (no error)=w181) -> (error out=w180:errorcluster)
            n59 = call <vilib>:"Add State(s) to Queue__jki_lib_state_machine.vi"("State(s) in (\"\")"=w184) -> ("States Out"=w183:string)  [unwired: 14 in]
          }
          frame "---------- UI ----------" {
            # "Do not put any code in this frame.\n(It is a separator no-op. You can make a copy of this frame to create a new UI frame)"
            n60 = call <vilib>:"Add State(s) to Queue__jki_lib_state_machine.vi"("State(s) in (\"\")"=w189) -> ("States Out"=w188:string)  [unwired: 14 in]
          }
          frame "UI: Initialize" {
            # "Initialize the User Interface, here.\n(this is called automatically, by the Macro: Init)"
            n61 = call <vilib>:"Add State(s) to Queue__jki_lib_state_machine.vi"("State(s) in (\"\")"=w194) -> ("States Out"=w193:string)  [unwired: 14 in]
          }
          frame "UI: Cursor Set" {
            # "Argument"
            # "Initialize the User Interface, here.\n(this is called automatically, by the Macro: Init)"
            n62 = disable-structure shown="Default" {
              disable-tunnel: w197 -> [w202 w205]
              disable-tunnel: [w202 w204] -> w196
              disable-tunnel: w195 -> [_ w203]
              frame condition #0 {
              }
              frame condition #1 (active) {
                n63 = case shown="\"Idle\", Default" w203 {
                  tunnel: w205 -> [w207 w209]
                  tunnel: [w206 w208] -> w204
                  frame "Idle", Default {
                    n64 = call <vilib>:"Unset Busy.vi"("error in (no error)"=w207) -> ("error out"=w206:errorcluster)  [unwired: 10 in]
                  }
                  frame "Busy" {
                    n65 = call <vilib>:"Set Busy.vi"("error in (no error)"=w209) -> ("error out"=w208:errorcluster)  [unwired: 9 in, 1 out]
                  }
                }
              }
            }
            n66 = call <vilib>:"Add State(s) to Queue__jki_lib_state_machine.vi"("State(s) in (\"\")"=w201) -> ("States Out"=w200:string)  [unwired: 14 in]
          }
          frame "UI: Front Panel State" {
            # "Argument"
            # "Set Front Panel Open or Closed\n(Usage: \"UI: Front Panel State >> Open|Close\")"
            n67 = Unbundle By Name(w213) -> ("Core.Current VI Reference"=w212:refnum<vi>)
            n68 = disable-structure shown="Default" {
              disable-tunnel: w215 -> [w221 w244]
              disable-tunnel: [w220 w244] -> w214
              disable-tunnel: w212 -> [w219 _]
              disable-tunnel: w211 -> [w218 _]
              frame condition #0 (active) {
                n69 = case shown="\"Open\", Default" w218 {
                  tunnel: w221 -> [w225 w238]
                  tunnel: [w227 w239] -> w220
                  tunnel: w219 -> [w226 w236]
                  frame "Open", Default {
                    n70 = property class="VI"(reference=w226, error in=w225) -> (reference out=w223:refnum<vi>, error out=w224:errorcluster, "FP.State"=w222:T7)
                    n71 = case shown="\"Closed\"" w222 {
                      tunnel: [w230 w233] -> w227
                      tunnel: w224 -> [w229 w233]
                      tunnel: w223 -> [w228 _]
                      frame "Closed" {
                        n72 = invoke class="VI" method="FP.Open"(reference=w228, error in=w229, "Activate"=TRUE, "State"=T7."Standard") -> (error out=w230:errorcluster)  [unwired: 1 in, 4 out]
                      }
                      frame Default {
                      }
                    }
                  }
                  frame "Close" {
                    n73 = property class="VI"(reference=w236, error in=w238) -> (reference out=w235:refnum<vi>, error out=w237:errorcluster, "FP.State"=w234:T7)
                    n74 = case shown="Default" w234 {
                      tunnel: [w240 w243] -> w239
                      tunnel: w237 -> [w240 w242]
                      tunnel: w235 -> [_ w241]
                      frame "Invalid", "Closed" {
                      }
                      frame Default {
                        n75 = invoke class="VI" method="FP.Close"(reference=w241, error in=w242) -> (error out=w243:errorcluster)  [unwired: 1 in, 2 out]
                      }
                    }
                  }
                }
              }
              frame condition #1 {
              }
            }
            n76 = call <vilib>:"Add State(s) to Queue__jki_lib_state_machine.vi"("State(s) in (\"\")"=w217) -> ("States Out"=w216:string)  [unwired: 14 in]
          }
          frame "---------- Macro ----------" {
            # "Do not put any code in this frame.\n(It is a separator no-op. You can make a copy of this frame to create a new Macro frame)"
            n77 = call <vilib>:"Add State(s) to Queue__jki_lib_state_machine.vi"("State(s) in (\"\")"=w249) -> ("States Out"=w248:string)  [unwired: 14 in]
          }
          frame "Macro: Initialize" {
            # "Initialization Macro\n(This is called once, when the VI starts)"
            n78 = call <vilib>:"Add State(s) to Queue__jki_lib_state_machine.vi"("State(s) in Front (\"\")"="Data: Initialize\nInitialize Core Data\nEvents: Register", "State(s) in (\"\")"="Process: Sync", "State(s) at Back (\"\")"="UI: Initialize\nUI: Front Panel State >> Open\nData: Register Stream") -> ("States Out"=w251:string)  [unwired: 12 in]
            n79 = call <vilib>:"Add State(s) to Queue__jki_lib_state_machine.vi"("State(s) in Front (\"\")"=w251, "State(s) in (\"\")"=w258) -> ("States Out"=w257:string)  [unwired: 13 in]
          }
          frame "Macro: Exit" {
            # "Exit Macro\n(This is called once, when the VI exits)"
            n80 = Unbundle By Name(w263) -> ("Core.Close Panel on Exit?"=w269:bool)
            n81 = Select(t="//UI: Front Panel State >> Close", s=w269, f="") -> (s? t:f=w266:string)
            n82 = call <vilib>:"Add State(s) to Queue__jki_lib_state_machine.vi"("State(s) in Front (\"\")"="USB4431: Shutdown\nData: Cleanup\nEvents: Unregister", "State(s) in (\"\")"="Process: Sync", "State(s) at Back (\"\")"="Exit") -> ("States Out"=w260:string)  [unwired: 12 in]
            n83 = call <vilib>:"Add State(s) to Queue__jki_lib_state_machine.vi"("State(s) in (\"\")"=w266, "State(s) at Back (\"\")"=w260) -> ("States Out"=w265:string)  [unwired: 13 in]
            n84 = call <vilib>:"Add State(s) to Queue__jki_lib_state_machine.vi"("State(s) in Front (\"\")"=w265, "State(s) in (\"\")"=w272) -> ("States Out"=w271:string)  [unwired: 13 in]
          }
          frame "---------- Process ----------" {
            # "Template Separator\n(You can make a copy of, or modify, this frame)"
            n85 = call <vilib>:"Add State(s) to Queue__jki_lib_state_machine.vi"("State(s) in (\"\")"=w277) -> ("States Out"=w276:string)  [unwired: 14 in]
          }
          frame "Process: Sync" {
            n86 = Unbundle By Name(w285) -> ("Self Reference"=w281:refnum<class "SynchIO.PXI-4461.lvclass">)
            n87 = disable-structure shown="Enabled" {
              disable-tunnel: [w292 FALSE ("Don't run?")] -> w284
              disable-tunnel: w281 -> [w291 _]
              disable-tunnel: w280 -> [w290 _]
              disable-tunnel: [w289 _] -> w279
              frame Enabled {
                n88 = call <vilib>:"WaitOnProcessSync.vi"("error in (no error)"=w290, "SMO"=w291) -> ("error out"=w289:errorcluster, "Don't run?"=w292:bool)  [unwired: 7 in, 1 out]
              }
              frame Disabled {
              }
            }
            n89 = Select(t="Data: Cleanup\nEvents: Unregister\nExit", s=w284, f="") -> (s? t:f=w278:string)
            n90 = call <vilib>:"Add State(s) to Queue__jki_lib_state_machine.vi"("State(s) in Front (\"\")"=w278, "State(s) in (\"\")"=w288) -> ("States Out"=w287:string)  [unwired: 13 in]
          }
          frame "---------- Events ----------" {
            # "Template Separator\n(You can make a copy of, or modify, this frame)"
            n91 = call <vilib>:"Add State(s) to Queue__jki_lib_state_machine.vi"("State(s) in (\"\")"=w298) -> ("States Out"=w297:string)  [unwired: 14 in]
          }
          frame "Events: Register" {
            # "Expand to add\nmore events"
            # "Self Events (API Calls)"
            # "Base Class Protected Events"
            n92 = Unbundle By Name(w309) -> ("Self Reference"=w304:refnum<class "SynchIO.PXI-4461.lvclass">)
            n93 = call <vilib>:"GetProtectedEvents.vi"("SMO"=w304) -> ("error out"=w300:errorcluster, "SMO Protected Events"=w307:T10, "SMO out"=w306:refnum<class "SynchIO.PXI-4461.lvclass">)  [unwired: 8 in]
            n94 = call "SynchIO.USB4431.GetProtectedEvents.vi"("SynchIO.USB4431"=w306) -> ("error out"=w301:errorcluster, "Protected Events"=w305:T11)  [unwired: 8 in, 1 out]
            n95 = register-events(w307, w305) -> (reference out=w308:refnum<event-registration>, error out=w302:errorcluster)  [unwired: 2 in]
            n96 = Merge Errors(w303, w302, w301, w300) -> (w299:errorcluster)
            n97 = call <vilib>:"Add State(s) to Queue__jki_lib_state_machine.vi"("State(s) in (\"\")"=w311) -> ("States Out"=w310:string)  [unwired: 14 in]
          }
          frame "Events: Unregister" {
            n98 = Unregister For Events(event registration refnum=w314, error in=w313) -> (error out=w312:errorcluster)
            n99 = call <vilib>:"Clear Errors.vi"("error in (no error)"=w312) -> ()  [unwired: 5 in, 2 out]
            n100 = call <vilib>:"Add State(s) to Queue__jki_lib_state_machine.vi"("State(s) in (\"\")"=w317) -> ("States Out"=w316:string)  [unwired: 14 in]
          }
          frame "---------- API ----------" {
            n101 = call <vilib>:"Add State(s) to Queue__jki_lib_state_machine.vi"("State(s) in (\"\")"=w322) -> ("States Out"=w321:string)  [unwired: 14 in]
          }
          frame "API: NewData" {
            n102 = Unbundle By Name(w327) -> ("Self Reference"=w326:refnum<class "SynchIO.PXI-4461.lvclass">, "Your string data"=w323:string)
            n103 = call "SynchIO.USB4431.SetData.vi"("error in (no error)"=w325, "Data In"=w323, "SynchIO.USB4431"=w326) -> ("error out"=w324:errorcluster)  [unwired: 7 in, 1 out]
            n104 = call <vilib>:"Add State(s) to Queue__jki_lib_state_machine.vi"("State(s) in (\"\")"=w330, "State(s) at Back (\"\")"=w323) -> ("States Out"=w329:string)  [unwired: 13 in]
          }
          frame "API: Initialize" {
            n105 = call <vilib>:"Add State(s) to Queue__jki_lib_state_machine.vi"("State(s) in (\"\")"=w335) -> ("States Out"=w334:string)  [unwired: 14 in]
          }
          frame "----------USB-4431---------- " {
            n106 = call <vilib>:"Add State(s) to Queue__jki_lib_state_machine.vi"("State(s) in (\"\")"=w340) -> ("States Out"=w339:string)  [unwired: 14 in]
          }
          frame "USB-4431: Initialize" {
            w342 = 10123 items=["Finite Samples"=10178, "Continuous Samples"=10123] ("sample mode")
            n107 = Unbundle By Name(w349) -> ("AI Buffer Size (S)"=w341:i32, "AI Configuration"=w353:T2, "AO Configuration"=w352:T3, "AO"=w351:T4, "sampling info"=w350:cluster{"Fs":dbl, "#s":dbl})
            n108 = call "4461 - Create IO Channels Parallel Uneven.vi"("sample mode"=w342, "error in"=w346, "AI Buffer Size (S)"=w341, "sampling info"=w350, "AO"=w351, "AO Configuration"=w352, "AI Configuration"=w353) -> ("AO Task"=w343:refnum<k21>[], "AI task"=w344:refnum<k21>[], "error out"=w345:errorcluster)  [unwired: 1 in, 1 out]
            n109 = Bundle By Name(cluster=w349, "AI task"=w344, "AO Task"=w343) -> (w348:T8)
            n110 = call <vilib>:"Add State(s) to Queue__jki_lib_state_machine.vi"("State(s) in Front (\"\")"="USB-4431: ReadWrite" ("message"), "State(s) in (\"\")"=w356) -> ("States Out"=w355:string)  [unwired: 13 in]
          }
          frame "USB-4431: ReadWrite" {
            n111 = Unbundle By Name(w370) -> ("AI task"=w363:refnum<k21>[], "AO Task"=w364:refnum<k21>[], "sampling info"=w368:cluster{"Fs":dbl, "#s":dbl}, "AO Data"=w362:waveform(dbl)[], "Iteration"=w357:i32)
            n112 = Equal To 0?(x=w357) -> (x = 0?=w359:bool)
            n113 = call "4461 - AI AND AI - Read AND Write Uneven.vi"("Reset"=w359, "AO Array"=w362, "error in (no error)"=w360, "sampling info"=w368, "AO Task"=w364, "AI task"=w363) -> ("error out"=w365:errorcluster, "Input Signals"=w367:waveform(dbl)[])  [unwired: 4 in]
            "Signals Graph" <- w367
            n114 = Increment(x=w357) -> (x+1=w358:i32)
            n115 = case shown="False" "stop" {
              tunnel: ["USB-4431: Publish" "USB-4431: Shutdown"] -> w366
              frame False {
              }
              frame True {
              }
            }
            n116 = Bundle By Name(cluster=w370, "AI Data"=w367, "Iteration"=w358) -> (w369:T8)
            n117 = call <vilib>:"Add State(s) to Queue__jki_lib_state_machine.vi"("State(s) in Front (\"\")"=w366, "State(s) in (\"\")"=w373) -> ("States Out"=w372:string)  [unwired: 13 in]
          }
          frame "USB-4431: Publish" {
            n118 = Unbundle By Name(w382) -> ("AI Data"=w376:waveform(dbl)[], "writer endpoint"=w378:refnum<k21>)
            n119 = shared-variable-write(w378, w376) -> (w377:refnum<k21>)  [unwired: 2 in, 2 out]
            n120 = Bundle By Name(cluster=w382, "AI Data"=w376, "writer endpoint"=w377) -> (w381:T8)
            n121 = call <vilib>:"Add State(s) to Queue__jki_lib_state_machine.vi"("State(s) in Front (\"\")"="USB-4431: ReadWrite", "State(s) in (\"\")"=w385) -> ("States Out"=w384:string)  [unwired: 13 in]
          }
          frame "USB-4431: Shutdown" {
            n122 = Unbundle By Name(w392) -> ("AI task"=w390:refnum<k21>[], "AO Task"=w389:refnum<k21>[], "writer endpoint"=w387:refnum<k21>)
            n123 = Build Array (concatenate)(w390, w389) -> (w388:refnum<k21>[])
            n124 = for {
              tunnel: [w400] -> w394
              tunnel: w393 -> [w399]
              tunnel: w388 -> [w398] mode=indexing
              n125 = flat-sequence {
                tunnel: [w405] -> w401
                tunnel: w399 -> [w404]
                tunnel: w398 -> [w403]
                tunnel: [w406] -> w402
                tunnel: w401 -> [w406]
                tunnel: w402 -> [w409]
                tunnel: [w408] -> w400
                frame #0 {
                  n126 = call <vilib>:"DAQmx Stop Task.vi"("task/channels in"=w403, "error in"=w404) -> ("task out"=w405:refnum<k21>)  [unwired: 12 in, 1 out]
                }
                frame #1 {
                  n127 = Wait (ms)(milliseconds to wait=u32 50) -> ()  [unwired: 1 out]
                }
                frame #2 {
                  n128 = call <vilib>:"DAQmx Clear Task.vi"("task in"=w409) -> ("error out"=w408:errorcluster)  [unwired: 14 in]
                }
                frame #3 {
                  n129 = Wait (ms)(milliseconds to wait=u32 50) -> ()  [unwired: 1 out]
                }
              }
            }
            n130 = Flush Stream(11:w387) -> (3:w386:refnum<k21>)  [unwired: 3 in, 2 out]
            n131 = Destroy Stream Endpoint(11:w386) -> ()  [unwired: 1 in, 1 out]
            n132 = call <vilib>:"Add State(s) to Queue__jki_lib_state_machine.vi"("State(s) in Front (\"\")"="Macro: Exit", "State(s) in (\"\")"=w397) -> ("States Out"=w396:string)  [unwired: 13 in]
          }
        }
        n133 = call "StateHistory.vi"("Current State in"=w16) -> ("Current State out"=→"Current State":string, "delimited string"=→"State History":string)  [unwired: 9 in]
      }
    }
    frame Error {
    }
  }
  n134 = call-parent "Process.vi"("error in"=w7, "SynchIO"=w6) -> ("error out"=w4:errorcluster, "SynchIO out"=→"SynchIO.USB4431 out":refnum<class "SynchIO.PXI-4461.lvclass">)  [unwired: 8 in]
  n135 = Merge Errors(w4, w3) -> (→"error out":errorcluster)
